vi "asset.property_value_at.vi"(8 "error in":errorcluster, 11 "object_in":refnum<class "Asset.lvclass">) -> (0 "error out":errorcluster, 3 "object_out":refnum<class "Asset.lvclass">)   [LabVIEW 2020, in "Asset.lvclass"]
doc: "Returns the value of the property at the given index."
uses:
  Asset.lvclass
  Asset.lvclass/Asset.ctl
  client.lvlib
panel:
  out "out_needed out":u32
  out "function return":i32
  out "buf out":string
  in  "index":i32
  in  "buf":string
  in  "cap":u32
  in  "out_needed":u32
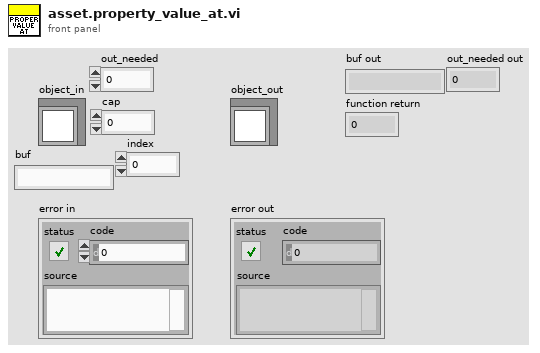
[diagram p1: front panel]
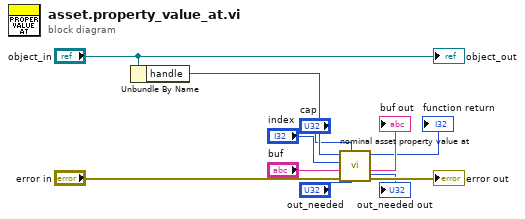
[diagram p0: block diagram]
diagram:
  n1 = Unbundle By Name("object_in") -> ("handle"=w9:i32)
  n2 = call "nominal asset property value at.vi"("out_needed"="out_needed", "cap"="cap", "error in (no error)"="error in", "buf"="buf", "index"="index", "asset"=w9) -> ("error out"=→"error out":errorcluster, "buf out"=→"buf out":string, "function return"=→"function return":i32, "out_needed out"=→"out_needed out":u32)  [unwired: 2 in]
  "object_out" <- "object_in"
